vi "http check to close connection.vi"(11 "application request":T1) -> (1 "leave connection open?":bool, 2 "stop process?":bool, 3 "application request out":T1)   [LabVIEW 2016, in "Basic HTTPS server.lvclass"]
uses:
  Basic HTTPS server.lvclass
  http response.ctl
  HTTP headers/http header data.ctl
  HTTP headers/http headers.lvlib
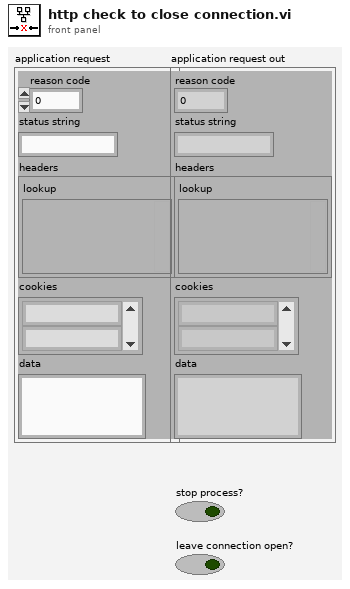
[diagram p1: front panel]
types:
  T1 = typedef "Basic HTTPS server.lvclass/http response.ctl" = cluster{"reason code":u16, "status string":string, "headers":T2, "cookies":string[], "data":string}
  T2 = typedef "http headers.lvlib/http header data.ctl" = cluster{"lookup":variant}
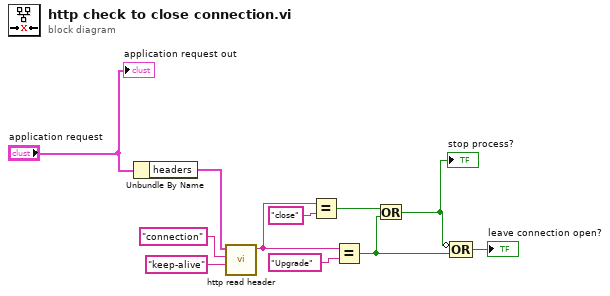
[diagram p0: block diagram]
diagram:
  n1 = Unbundle By Name("application request") -> ("headers"=w4:T2)
  n2 = call "http read header.vi"("default value"="keep-alive", "header field name"="connection" ("name"), "headers"=w4) -> ("value"=w1:string)  [unwired: 7 in, 1 out]
  n3 = Equal?(x=w1, y="close" ("name")) -> (x = y?=w7:bool)
  n4 = Equal?(x=w1, y="Upgrade" ("name")) -> (x = y?=w8:bool)
  n5 = Or(x=w7, y=w8) -> (x .or. y?=w9:bool)
  "stop process?" <- w9
  n6 = Compound Arithmetic op=OR(invert w9, w8) -> (→"leave connection open?":bool)
  "application request out" <- "application request"
